vi "Variant to Array.vi"(8 "error in (no error)":errorcluster, 11 "Data (Variant)":variant) -> (0 "error out":errorcluster, 2 "2D Array":dbl[][](array[numeric]), 3 "1D Array":dbl[](array[numeric]))   [LabVIEW 2016, in "Data.lvclass"]
uses:
  Data.lvclass
  <vilib>/Utility/error.llb/Error Cluster From Error Code.vi
  <vilib>/ErrorRing/Error Ring.xnode
  <vilib>/Utility/Data Type/NI_Data Type.lvlib
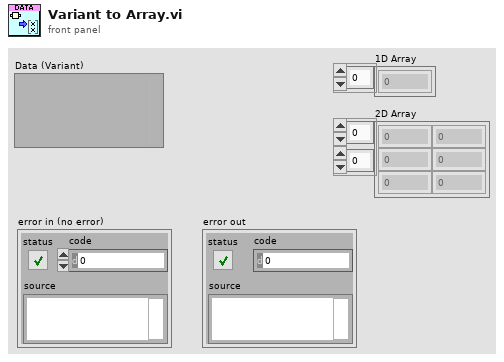
[diagram p1: front panel]
types:
  T1 = typedef "NI_Data Type.lvlib/Data Type.ctl" = enum8{"Invalid Type", "Void", "I8", "I16", "I32", "I64", "U8", "U16", "U32", "U64", "Single Float", "Double Float", "Extended Float", "Single Complex", "Double Complex", "Extended Complex", "Enum U8", "Enum U16", "Enum U32", "Enum U64", "Single Float With Unit", "Double Float With Unit", "Extended Float With Unit", "Single Complex with Unit", "Double Complex with Unit", "Extended Complex with Unit", "Boolean", "String", "Path", "Picture", "Tag", "Array", "Cluster", "Variant", "LV Variant", "Waveform", "Timestamp", "Digital Waveform", "Digital Data", "ExpressData", "Refnum", "External Data", "VI", "Poly VI", "LabVIEW Class Instance", "Fixed Point"}
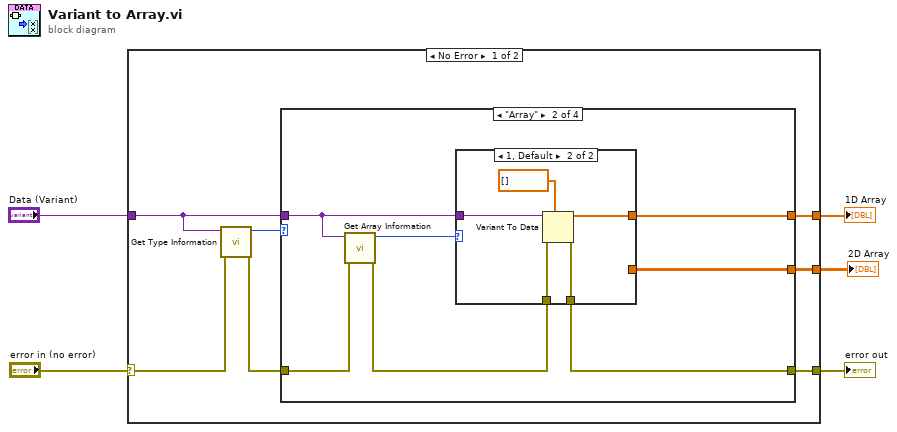
[diagram p0: block diagram]
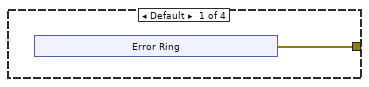
[diagram p2: hidden frame]
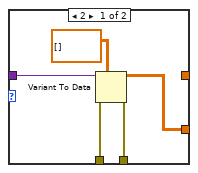
[diagram p3: hidden frame]
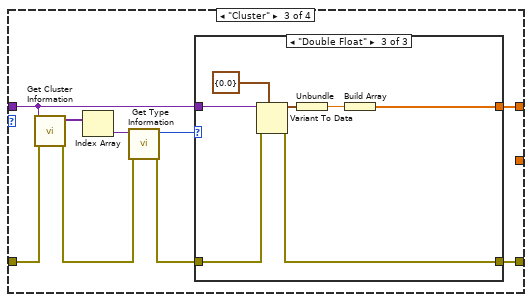
[diagram p4: hidden frame]
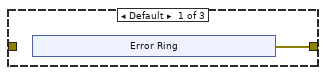
[diagram p5: hidden frame]
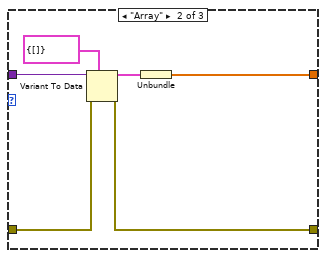
[diagram p6: hidden frame]
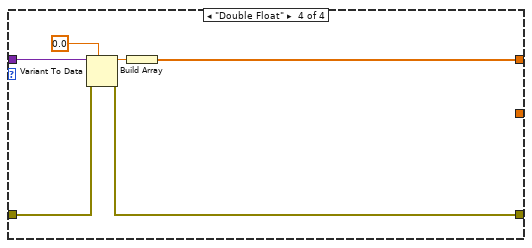
[diagram p7: hidden frame]
diagram:
  n1 = case shown="No Error" "error in (no error)" {
    selector: "error in (no error)" -> [w7 w68]
    tunnel: [w11 _] -> w5
    tunnel: [w8 w68] -> w4
    tunnel: "Data (Variant)" -> [w10 _]
    tunnel: [w6 _] -> w1
    frame No Error {
      n2 = call <vilib>:"Get Type Information.vi"("error in (no error)"=w7, "Variant"=w10) -> ("error out"=w9:errorcluster, "Type"=w12:T1)  [unwired: 5 in, 3 out]
      n3 = case shown="\"Array\"" w12 {
        tunnel: [w13 w24 w38 w62] -> w8
        tunnel: [_ w19 w35 w64] -> w11
        tunnel: w10 -> [_ w23 w36 w66]
        tunnel: w9 -> [_ w22 w43 w63]
        tunnel: [_ w18 _ _] -> w6
        frame Default {
          n4 = xnode "Error Ring"() -> ("error out"=w13:errorcluster)
        }
        frame "Array" {
          n5 = call <vilib>:"Get Array Information.vi"("error in (no error)"=w22, "Variant"=w23) -> ("error out"=w21:errorcluster, "Number of Dimensions"=w20:i32)  [unwired: 6 in, 2 out]
          n6 = case shown="1, Default" w20 {
            tunnel: [w28 w33] -> w24
            tunnel: w23 -> [w27 w32]
            tunnel: w21 -> [w26 w31]
            tunnel: [_ w30] -> w19
            tunnel: [w25 _] -> w18
            frame 2 {
              n7 = Variant To Data(error in=w26, type=dbl[][] [], Variant=w27) -> (data=w25:dbl[][], error out=w28:errorcluster)
            }
            frame 1, Default {
              n8 = Variant To Data(error in=w31, type=dbl[] [], Variant=w32) -> (data=w30:dbl[], error out=w33:errorcluster)
            }
          }
        }
        frame "Cluster" {
          n9 = call <vilib>:"Get Cluster Information.vi"("error in (no error)"=w43, "Variant"=w36) -> ("error out"=w40:errorcluster, "Cluster Elements"=w42:variant[])  [unwired: 8 in]
          n10 = Index Array(array=w42) -> (element=w41:variant)  [unwired: 1 in]
          n11 = call <vilib>:"Get Type Information.vi"("error in (no error)"=w40, "Variant"=w41) -> ("error out"=w39:errorcluster, "Type"=w37:T1)  [unwired: 5 in, 3 out]
          n12 = case shown="\"Double Float\"" w37 {
            tunnel: [w44 w52 w58] -> w38
            tunnel: [_ w50 w60] -> w35
            tunnel: w39 -> [_ w53 w59]
            tunnel: w36 -> [_ w49 w55]
            frame Default {
              n13 = xnode "Error Ring"() -> ("error out"=w44:errorcluster)
            }
            frame "Array" {
              n14 = Variant To Data(error in=w53, type=cluster{dbl[]} {[]}, Variant=w49) -> (data=w54:cluster{dbl[]}, error out=w52:errorcluster)
              n15 = Unbundle(w54) -> (w50:dbl[])
            }
            frame "Double Float" {
              n16 = Variant To Data(error in=w59, type=cluster{dbl} {0.0}, Variant=w55) -> (data=w61:cluster{dbl}, error out=w58:errorcluster)
              n17 = Unbundle(w61) -> (w56:dbl)
              n18 = Build Array(w56) -> (w60:dbl[])
            }
          }
        }
        frame "Double Float" {
          n19 = Variant To Data(error in=w63, type=0.0, Variant=w66) -> (data=w67:dbl, error out=w62:errorcluster)
          n20 = Build Array(w67) -> (w64:dbl[])
        }
      }
    }
    frame Error {
    }
  }
  "1D Array" <- w5
  "error out" <- w4
  "2D Array" <- w1
